vi "32bit_to_bitstreamV2.vi"(6 "error in (no error)":errorcluster, 9 "24-bit pixmap":u32[][](array[numeric])) -> (0 "error out":errorcluster, 3 "Bitstream with Guard":u8[](array[numeric]))   [LabVIEW 2013]
panel:
  out "element":i32
  out "size(s)":i32
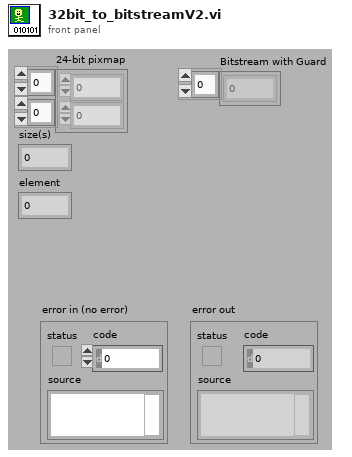
[diagram p1: front panel]
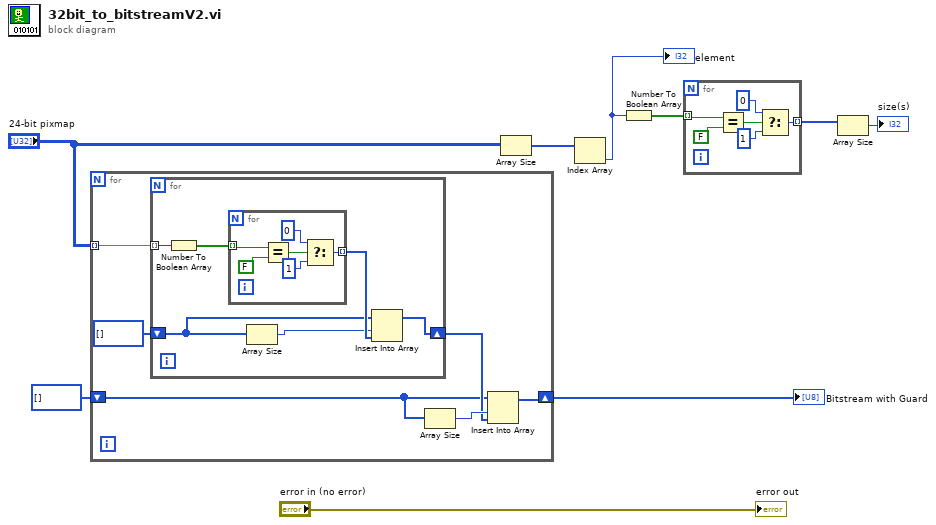
[diagram p0: block diagram]
diagram:
  n1 = for {
    tunnel: "24-bit pixmap" -> [w15] mode=indexing
    shift-right: [w12] -> w1
    shift-left: u8[] [] -> [w10]
    n2 = for {
      tunnel: w15 -> [w21] mode=indexing
      shift-right: [w19] -> w11
      shift-left: u8[] [] -> [w17]
      n3 = Number To Boolean Array(number=w21) -> (Boolean array=w16:bool[])
      n4 = for {
        tunnel: w16 -> [w27] mode=indexing
        tunnel: [w22] -> w20 mode=indexing
        n5 = Equal?(x=w27, y=FALSE) -> (x = y?=w25:bool)
        n6 = Select(t=u8 0, s=w25, f=u8 1) -> (s? t:f=w22:u8)
      }
      n7 = Array Size(array=w17) -> (size(s)=w18:i32)
      n8 = Insert Into Array(array=w17, index=w18, new element=w20) -> (w19:u8[])
    }
    n9 = Array Size(array=w10) -> (size(s)=w13:i32)
    n10 = Insert Into Array(array=w10, index=w13, new element=w11) -> (w12:u8[])
  }
  "Bitstream with Guard" <- w1
  n11 = Array Size(array="24-bit pixmap") -> (size(s)=w6:i32[])
  n12 = Index Array(array=w6) -> (element=w5:i32)  [unwired: 1 in]
  "element" <- w5
  n13 = Number To Boolean Array(number=w5) -> (Boolean array=w7:bool[])
  n14 = for {
    tunnel: w7 -> [w33] mode=indexing
    tunnel: [w28] -> w3 mode=indexing
    n15 = Equal?(x=w33, y=FALSE) -> (x = y?=w31:bool)
    n16 = Select(t=u8 0, s=w31, f=u8 1) -> (s? t:f=w28:u8)
  }
  n17 = Array Size(array=w3) -> (size(s)=→"size(s)":i32)
  "error out" <- "error in (no error)"
